vi "Initialize SV Interface.vi"(8 "error in (no error)":errorcluster, 11 "Process Data":T2={"Write URLs"={"URLs"=[]}, "Read URLs"={"URLs"=[]}, "Write SV FIFO"="", "Read SV FIFO"="", "Status SV FIFO"="", "Status Notifier"="", "Update Rate"=10}) -> (0 "error out":errorcluster, 3 "SV Data":T1={"Status notifier"=refnum, "Write FIFO ref"=refnum, "Read FIFO ref"=refnum, "Status FIFO ref"=refnum, "Update Rate"=1, "Write Refs by Type"={"DBL Write"=[]}, "Read Refs by Type"={"DBL Read"=[]}, "WriteSize"=0, "ReadSize"=0})   [LabVIEW 2020, in "Shared Variable Interface.lvlib"]
uses:
  Shared Variable Interface.lvlib
  Shared DataTypes/SV Process Data.ctl
  Shared DataTypes/URLs.ctl
  SV Process Configuration.ctl
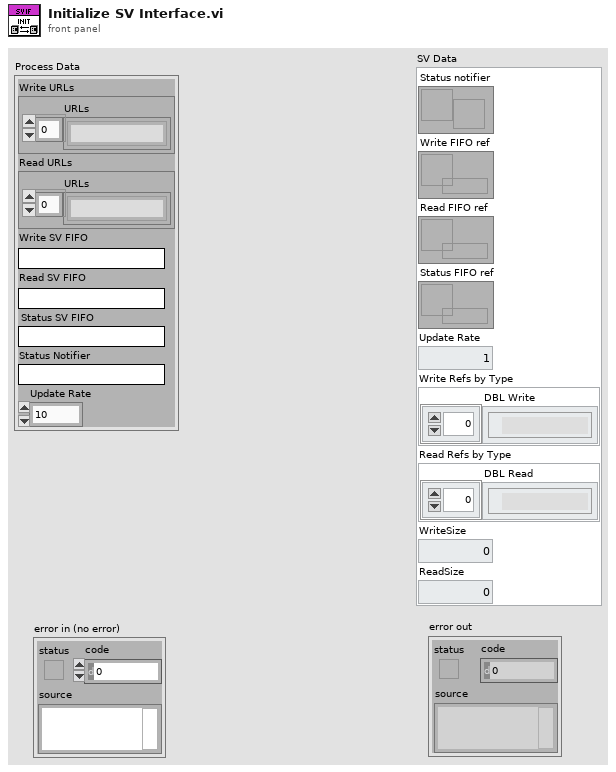
[diagram p1: front panel]
types:
  T1 = typedef "Shared Variable Interface.lvlib/SV Process Configuration.ctl" = cluster{"Status notifier":refnum<notifier>, "Write FIFO ref":refnum<k33>, "Read FIFO ref":refnum<k33>, "Status FIFO ref":refnum<k33>, "Update Rate":u32, "Write Refs by Type":cluster{"DBL Write":refnum<k21>[]}, "Read Refs by Type":cluster{"DBL Read":refnum<k21>[]}, "WriteSize":i32, "ReadSize":i32}
  T2 = typedef "SV Process Data.ctl" = cluster{"Write URLs":T3, "Read URLs":T3, "Write SV FIFO":string, "Read SV FIFO":string, "Status SV FIFO":string, "Status Notifier":string, "Update Rate":u32}
  T3 = typedef "URLs.ctl" = cluster{"URLs":string[]}
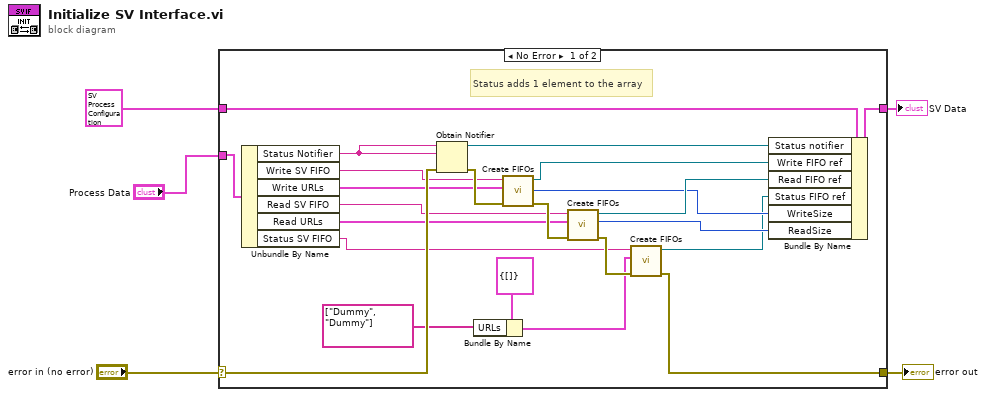
[diagram p0: block diagram]
diagram:
  n1 = case shown="No Error" "error in (no error)" {
    selector: "error in (no error)" -> [w27 w30]
    tunnel: [w7 w30] -> w4
    tunnel: [w24 w29] -> w1
    tunnel: T1 {"Status notifier"=refnum, "Write FIFO ref"=refnum, "Read FIFO ref"=refnum, "Status FIFO ref"=refnum, "Update Rate"=1, "Write Refs by Type"={"DBL Write"=[]}, "Read Refs by Type"={"DBL Read"=[]}, "WriteSize"=0, "ReadSize"=0} ("SV Data") -> [w25 w29]
    tunnel: "Process Data" -> [w22 _]
    frame No Error {
      # "Status adds 1 element to the array"
      n2 = Unbundle By Name(w22) -> ("Status Notifier"=w28:string, "Write SV FIFO"=w18:string, "Write URLs"=w21:T3, "Read SV FIFO"=w17:string, "Read URLs"=w19:T3, "Status SV FIFO"=w11:string)
      n3 = Obtain Notifier(name (unnamed)=w28, notification data type=w28, error in (no error)=w27) -> (notifier out=w23:refnum<notifier>, error out=w26:errorcluster)  [unwired: 1 in, 1 out]
      n4 = Bundle By Name(cluster=T3 {"URLs"=[]} ("URL Cluster"), "URLs"=string[] ["Dummy", "Dummy"]) -> (w9:T3)
      n5 = call "Create FIFOs.vi"("error in (no error)"=w26, "URL Cluster"=w21, "SV FIFO Name"=w18) -> ("error out"=w20:errorcluster, "size"=w14:i32, "FIFO ref"=w16:refnum<k33>)  [unwired: 6 in]
      n6 = call "Create FIFOs.vi"("error in (no error)"=w20, "URL Cluster"=w19, "SV FIFO Name"=w17) -> ("error out"=w12:errorcluster, "size"=w13:i32, "FIFO ref"=w15:refnum<k33>)  [unwired: 6 in]
      n7 = call "Create FIFOs.vi"("error in (no error)"=w12, "URL Cluster"=w9, "SV FIFO Name"=w11) -> ("error out"=w7:errorcluster, "FIFO ref"=w8:refnum<k33>)  [unwired: 6 in, 1 out]
      n8 = Bundle By Name(cluster=w25, "Status notifier"=w23, "Write FIFO ref"=w16, "Read FIFO ref"=w15, "Status FIFO ref"=w8, "WriteSize"=w14, "ReadSize"=w13) -> (w24:T1)
    }
    frame Error {
    }
  }
  "error out" <- w4
  "SV Data" <- w1
